vi "VirtualChannelTypes.vi"() -> (3 "Array":string[](array[string]))   [LabVIEW 2017, in "CmsVirtualChannel.lvlib"]
uses:
  <vilib>/addons/InsightCM/Devices/Shared/Cms/CmsVirtualChannel/CmsVirtualChannel.lvlib
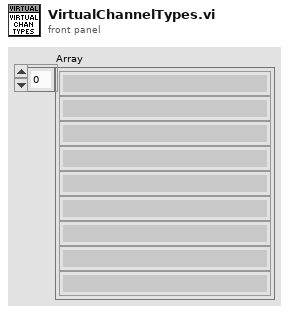
[diagram p1: front panel]
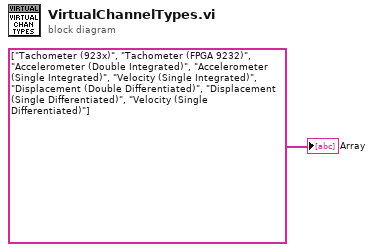
[diagram p0: block diagram]
diagram:
  "Array" <- string[] ["Tachometer (923x)", "Tachometer (FPGA 9232)", "Accelerometer (Double Integrated)", "Accelerometer (Single Integrated)", "Velocity (Single Integrated)", "Displacement (Double Differentiated)", "Displacement (Single Differentiated)", "Velocity (Single Differentiated)"] ("Array")
